vi "data_types_example_1.vi"() -> ()   [LabVIEW 2024]
panel:
  in  "Waveform Graph 2":dbl[](graph)
  out "Array 2":dbl[](array[numeric])
  in  "Array":dbl[](array[numeric])
  out "Waveform Graph":dbl[](graph)
  out "String 2":string
  in  "String":string
  out "Boolean 2":bool
  out "Floating Point2":dbl
  out "Integer2":i64
  in  "Boolean":bool
  in  "Floating Point":dbl
  in  "Integer":i64
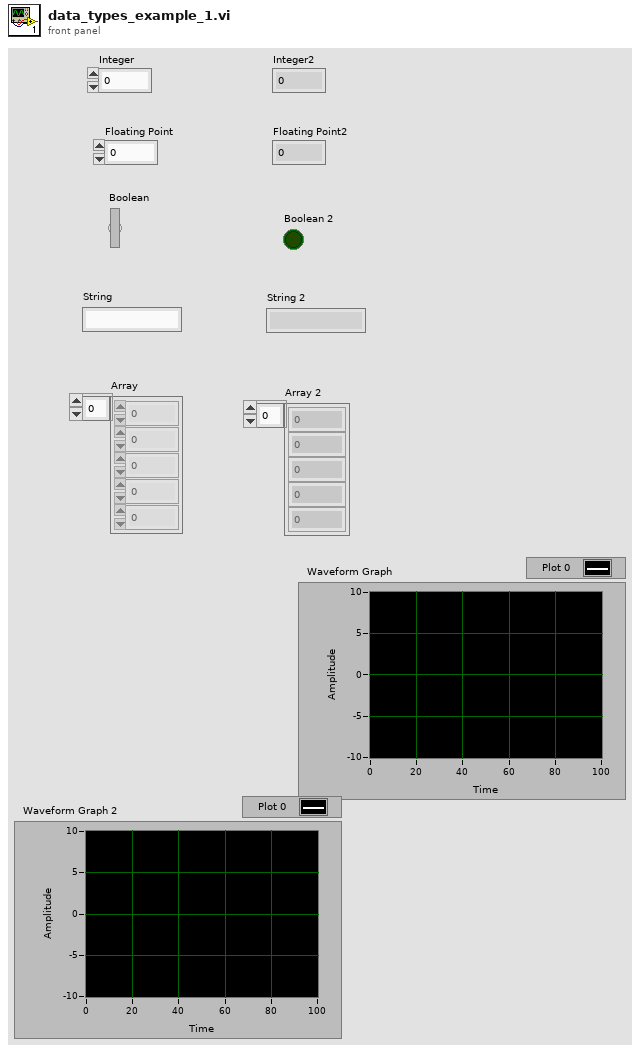
[diagram p1: front panel]
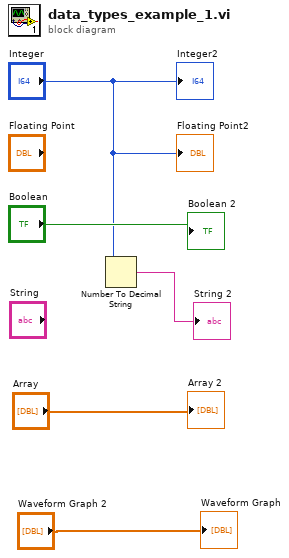
[diagram p0: block diagram]
diagram:
  n1 = Number To Decimal String(number="Integer") -> (decimal integer string=→"String 2":string)  [unwired: 1 in]
  "Integer2" <- "Integer"
  "Floating Point2" <- "Integer"
  "Boolean 2" <- "Boolean"
  "Waveform Graph" <- "Waveform Graph 2"
  "Array 2" <- "Array"
